vi "FlushValve.vi"() -> ()   [LabVIEW 2010]
panel:
  in  "Period (ms)":u32=500
  in  "Switches":i32=125
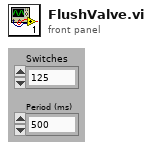
[diagram p1: front panel]
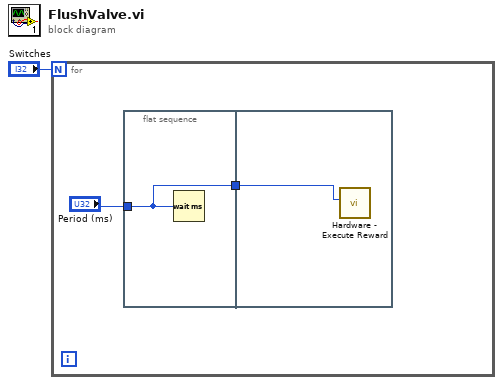
[diagram p0: block diagram]
diagram:
  n1 = for {
    N: "Switches" -> [_]
    n2 = flat-sequence {
      tunnel: "Period (ms)" -> [w4]
      tunnel: [w4] -> w2
      tunnel: w2 -> [w5]
      frame #0 {
        n3 = Wait (ms)(milliseconds to wait=w4) -> ()  [unwired: 1 out]
      }
      frame #1 {
        n4 = call "Hardware - Execute Reward.vi"("Reward Time (200 ms)"=w5) -> ()  [unwired: 10 in, 1 out]
      }
    }
  }
